vi "CLD3 FGV Timer no pause front panel.vi"(8 "error in (no error)":errorcluster, 10 "Wait":dbl, 11 "Timer Task":T1) -> (0 "error out":errorcluster, 2 "Time elapsed?":bool, 3 "Elapsed Time":dbl)   [LabVIEW 2009]
doc: "CLD 3 Challenge Exercise"
uses:
  CLD3 Timer Mode.ctl
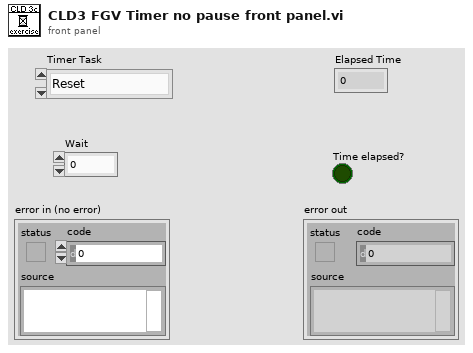
[diagram p1: front panel]
types:
  T1 = typedef "CLD3 Timer Mode.ctl" = enum16{"Reset", "Elapsed"}
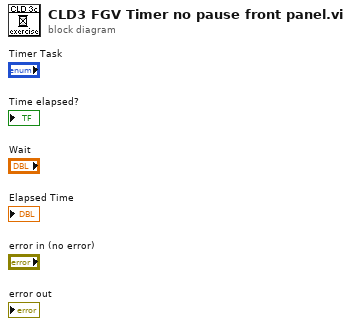
[diagram p0: block diagram]
diagram:
